vi "Send and Receive Message.vi"(6 "timeout (ms) [500]":i32=500, 8 "error in (no error)":errorcluster, 9 "Data":variant, 10 "Command":string, 11 "RemoteControl in":refnum<class "RemoteControl.lvclass">) -> (0 "error out":errorcluster, 1 "Data out":variant, 2 "Command out":string, 3 "RemoteControl out":refnum<class "RemoteControl.lvclass">)   [LabVIEW 2019, in "RemoteControl.lvclass"]
uses:
  RemoteControl.lvclass
  RemoteControl.lvclass/RemoteControl.ctl
panel:
  out "ID":string
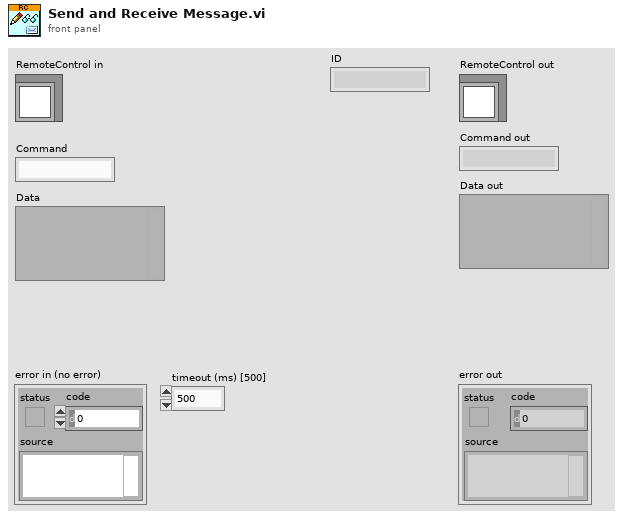
[diagram p1: front panel]
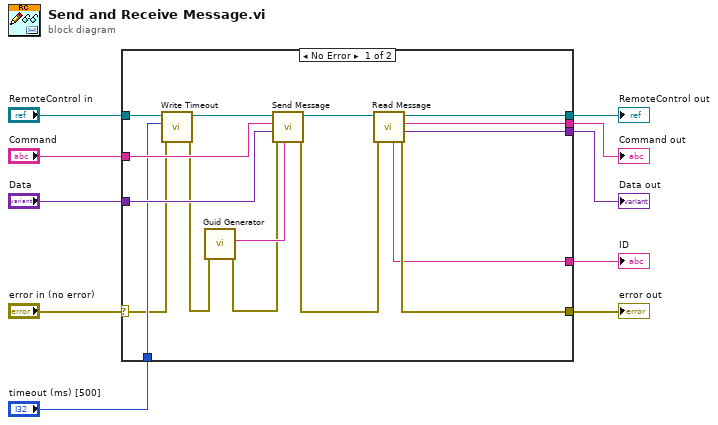
[diagram p0: block diagram]
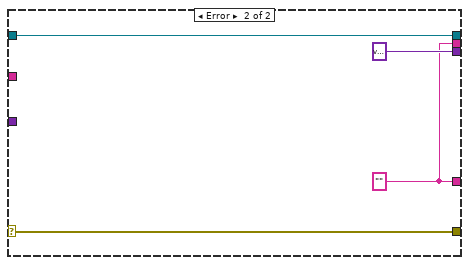
[diagram p2: hidden frame]
diagram:
  n1 = case shown="No Error" "error in (no error)" {
    selector: "error in (no error)" -> [w13 w30]
    tunnel: [w21 w30] -> w10
    tunnel: [w25 w29] -> w8
    tunnel: "RemoteControl in" -> [w15 w29]
    tunnel: "Command" -> [w19 _]
    tunnel: "Data" -> [w24 _]
    tunnel: [w23 w27] -> w5
    tunnel: [w22 variant ("Data")] -> w4
    tunnel: [w17 w27] -> w3
    tunnel: "timeout (ms) [500]" -> [w16 _]
    frame No Error {
      n2 = call "Write Timeout.vi"("error in (no error)"=w13, "timeout (ms) [500]"=w16, "RemoteControl in"=w15) -> ("error out"=w12:errorcluster, "RemoteControl out"=w14:refnum<class "RemoteControl.lvclass">)  [unwired: 7 in]
      n3 = call <vilib>:"Guid Generator.vi"("error in (no error)"=w12) -> ("error out"=w11:errorcluster, "GUID"=w18:string)  [unwired: 9 in]
      n4 = call-dynamic "Send Message.vi"("ID"=w18, "error in (no error)"=w11, "Data"=w24, "Command"=w19, "RemoteControl in"=w14) -> ("error out"=w20:errorcluster, "RemoteControl out"=w26:refnum<class "RemoteControl.lvclass">)  [unwired: 5 in]
      n5 = call-dynamic "Read Message.vi"("error in (no error)"=w20, "RemoteControl in"=w26) -> ("error out"=w21:errorcluster, "Data"=w22:variant, "Command"=w23:string, "RemoteControl out"=w25:refnum<class "RemoteControl.lvclass">, "ID"=w17:string)  [unwired: 5 in]
    }
    frame Error {
      w27 = "" ("Command")
    }
  }
  "error out" <- w10
  "RemoteControl out" <- w8
  "Command out" <- w5
  "Data out" <- w4
  "ID" <- w3
